vi "Configure Sequencer List Signal.vi"(7 "Signal (\"CW\")":string="CW", 8 "error in (no error)":errorcluster, 9 "Index (0)":i32, 10 "Instance (1)":i32=1, 11 "VISA resource name":refnum<visa-resource-name>) -> (0 "error out":errorcluster, 3 "VISA resource name out":refnum<visa-resource-name>)   [LabVIEW 2015, in "Rohde&Schwarz CMXP GPRF.lvlib"]
doc: "Defines the signal type for the sequencer list entry with the selected Index.\n\nAttribute:\nRSCMXPGPRF_ATTR_SEQUENCER_LIST_SIGNAL\n\nRemote-control command:\nSOURce:GPRF:GEN<i>:SEQuencer:LIST:SIGNal"
uses:
  <instrlib>/Rohde&Schwarz CMXP GPRF/Rohde&Schwarz CMXP GPRF.lvlib
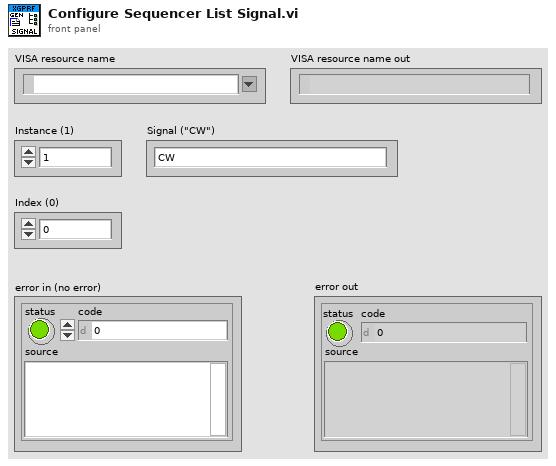
[diagram p1: front panel]
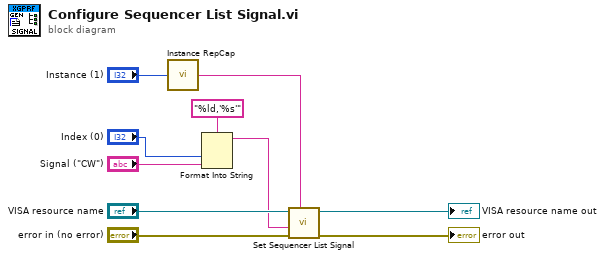
[diagram p0: block diagram]
diagram:
  n1 = call <instrlib>:"Instance RepCap.vi"("instance  in"="Instance (1)") -> ("instance out"=w10:string)
  n2 = Format Into String(format string="%ld,'%s'", "Index (0)", "Signal (\"CW\")") -> (resulting string=w1:string)  [unwired: 2 in, 1 out]
  n3 = call "Set Sequencer List Signal"("Repeated Capabilities"=w10, "error in (no error)"="error in (no error)", "Sequencer List Signal ()"=w1, "instrument handle"="VISA resource name") -> ("error out"=→"error out":errorcluster, "instrument handle out"=→"VISA resource name out":refnum<visa-resource-name>)  [unwired: 6 in]
